vi "AlliGator Check Invalid Python Plugin Input Parameter Types.vi"(8 "error in (no error)":errorcluster, 9 "Source":string, 11 "Invalid Parameter Types":string[](array[string])) -> (0 "error out":errorcluster)   [LabVIEW 2021, in "AlliGator Python Plugins.lvlib"]
doc: "Formats error with invalid input parameter message."
uses:
  <vilib>/Utility/error.llb/Error Cluster From Error Code.vi
  <vilib>/ErrorRing/Error Ring.xnode
  AlliGator Python Plugins.lvlib
  Strings/Strings.lvlib
panel:
  # "see the AlliGator License on the block diagram (Ctrl+E or Window:Show Block Diagram)"
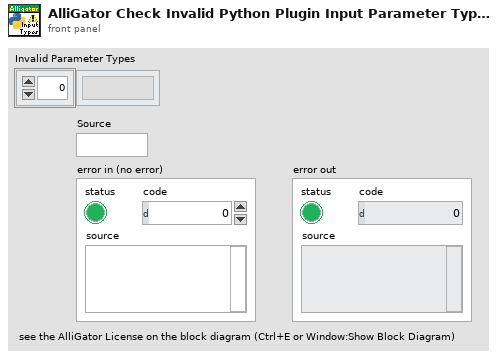
[diagram p1: front panel]
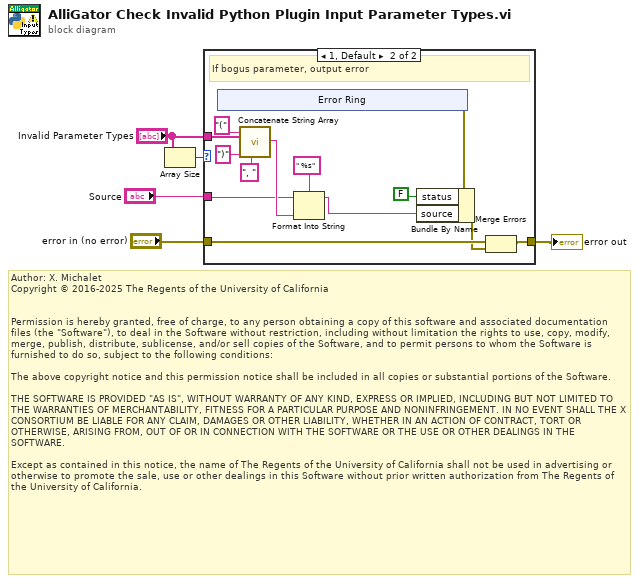
[diagram p0: block diagram]
diagram:
  # "Author: X. Michalet\nCopyright © 2016-2025 The Regents of the University of California\n \n\nPermission is hereby granted, free of charge, to any person obtaining a copy of this software and associated documentation files (the \"Software\"), to deal in the Software without restriction, including without limitation the rights to use, copy, modify, merge, publish, distribute, sublicense, and/or sell copies of the Software, and to permit persons to whom the Software is furnished to do so, subject to the following conditions:\n\nThe above copyright notice and this permission notice shall be included in all copies or substantial portions of the Software.\n\nTHE SOFTWARE IS PROVIDED \"AS IS\", WITHOUT WARRANTY OF ANY KIND, EXPRESS OR IMPLIED, INCLUDING BUT NOT LIMITED TO THE WARRANTIES OF MERCHANTABILITY, FITNESS FOR A PARTICULAR PURPOSE AND NONINFRINGEMENT. IN NO EVENT SHALL THE X CONSORTIUM BE LIABLE FOR ANY CLAIM, DAMAGES OR OTHER LIABILITY, WHETHER IN AN ACTION OF CONTRACT, TORT OR OTHERWISE, ARISING FROM, OUT OF OR IN CONNECTION WITH THE SOFTWARE OR THE USE OR OTHER DEALINGS IN THE SOFTWARE.\n\nExcept as contained in this notice, the name of The Regents of the University of California shall not be used in advertising or otherwise to promote the sale, use or other dealings in this Software without prior written authorization from The Regents of the University of California."
  n1 = Array Size(array="Invalid Parameter Types") -> (size(s)=w3:i32)
  n2 = case shown="1, Default" w3 {
    tunnel: "Invalid Parameter Types" -> [_ w19]
    tunnel: "error in (no error)" -> [w6 w16]
    tunnel: [w6 w17] -> w5
    tunnel: "Source" -> [_ w11]
    frame 0 {
    }
    frame 1, Default {
      # "If bogus parameter, output error"
      n3 = xnode "Error Ring"() -> ("error out"=w8:errorcluster)
      n4 = call "Concatenate String Array.vi"("Separator (TAB)"=", ", "Suffix (\"\")"=")" ("Suffix (\"\")"), "String Array"=w19, "Prefix (\"\")"="(" ("Prefix (\"\")")) -> ("Formatted String"=w15:string)  [unwired: 7 in]
      n5 = Format Into String(format string=" %s", initial string=w11, w15) -> (resulting string=w9:string)  [unwired: 1 in, 1 out]
      n6 = Bundle By Name(cluster=w8, "status"=FALSE, "source"=w9) -> (w7:errorcluster)
      n7 = Merge Errors(w16, w7) -> (w17:errorcluster)
    }
  }
  "error out" <- w5
